vi "close.vi"(2 "handle":i32, 3 "Error In":errorcluster caption="错误输入") -> (0 "return":i32, 1 "Error Out":errorcluster caption="错误输出")   [LabVIEW 2013, in "EM_CVx.lvlib"]
uses:
  EM_CVx.lvlib
  library/moverLibrary_x86.dll
  library/moverLibrary_x64.dll
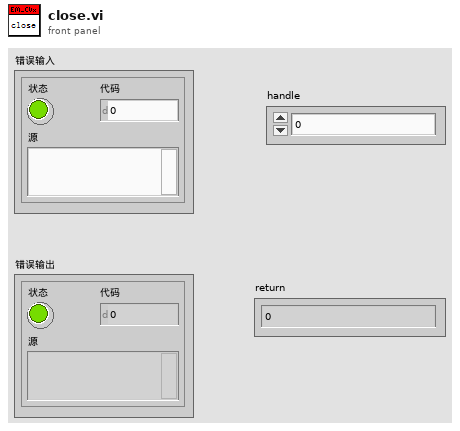
[diagram p1: front panel]
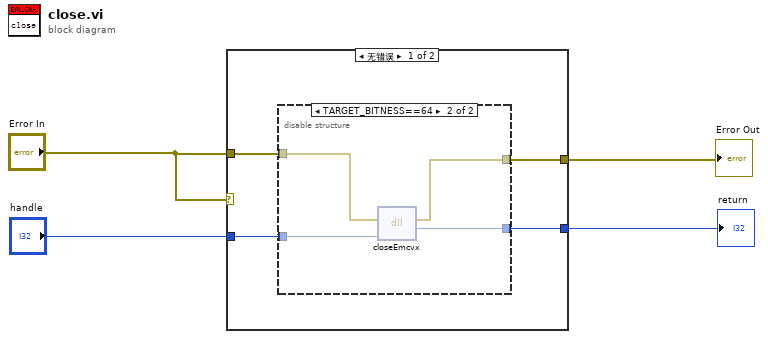
[diagram p0: block diagram]
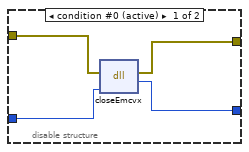
[diagram p2: hidden frame]
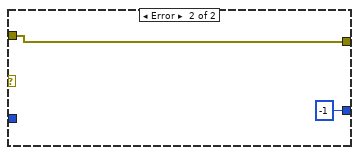
[diagram p3: hidden frame]
diagram:
  n1 = case shown="无错误" "Error In" {
    tunnel: "Error In" -> [w8 w18]
    tunnel: "handle" -> [w7 _]
    tunnel: [w6 w18] -> w3
    tunnel: [w5 -1 ("return")] -> w2
    frame No Error {
      n2 = disable-structure shown="TARGET_BITNESS==64" {
        disable-tunnel: w8 -> [w12 w16]
        disable-tunnel: w7 -> [w9 w15]
        disable-tunnel: [w11 w14] -> w6
        disable-tunnel: [w10 w13] -> w5
        frame condition #0 (active) {
          n3 = dll-call lib="E:/5-mover/4-labView/EM_CVx_2013/library/moverLibrary_x86.dll" fn="closeEmcvx"(error in=w12, "hdl"=w9) -> (error out=w11:errorcluster, "return"=w10:i32)  [unwired: 3 in, 1 out]
        }
        frame condition #1 {
          n4 = dll-call lib="E:/5-mover/4-labView/EM_CVx_2013/library/moverLibrary_x64.dll" fn="closeEmcvx"(error in=w16, "hdl"=w15) -> (error out=w14:errorcluster, "return"=w13:i32)  [unwired: 3 in, 1 out]
        }
      }
    }
    frame Error {
    }
  }
  "Error Out" <- w3
  "return" <- w2
